vi "Selectively clear model queue.vi"(7 "Queue clearing option":T2, 8 "error in (no error)":errorcluster, 11 "State(s) to look for [One per line]":string) -> (0 "error out":errorcluster, 3 "Cleared states":T1[](array[typedef]))   [LabVIEW 2018]
doc: "Get the queue reference and acts upon what is stored in it according to the \"Queue clearing option\" input.\n\nThe \"State(s) to look for\" input is the same format as the input for the \"Enqueue many states to controller\" VI. Meaning that it should be case-insensitive strings that name case(s), one per line, that pertain to the selected clearing option.\n\n\"Clear entire queue\" removes all pending states.\n\"Clear all that match\" removes all states, then re-queues states that don't match any of the ones in the input list.\n\"Clear all that don't match\" removes all states, then re-queues states that match one of the ones in the input list.\n\"Clear one of each match\" removes all states, then re-queues states that don't match the input list, but the input list only removes exactly one state per matching entry. This can be used to remove the first state that matches but leave the rest."
uses:
  Selective queue clearing methods.ctl
  Model queue data.ctl
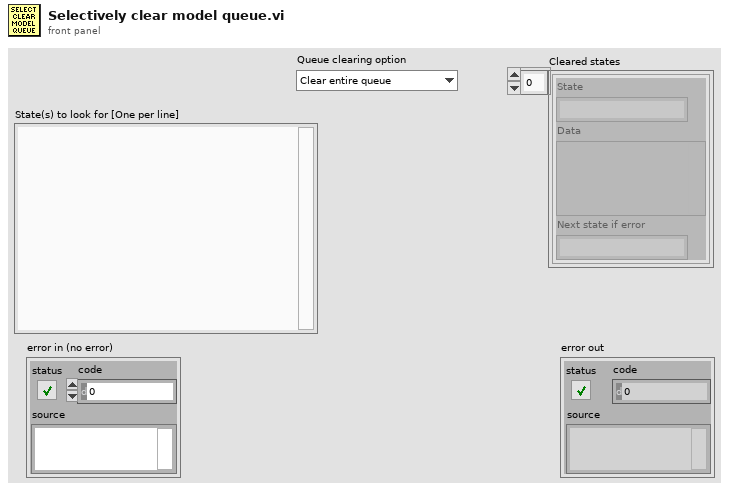
[diagram p1: front panel]
types:
  T1 = typedef "Model queue data.ctl" = cluster{"State":string, "Data":variant, "Next state if error":string}
  T2 = typedef "Selective queue clearing methods.ctl" = enum16{"Clear entire queue", "Clear all that match", "Clear all that don't match", "Clear one of each match"}
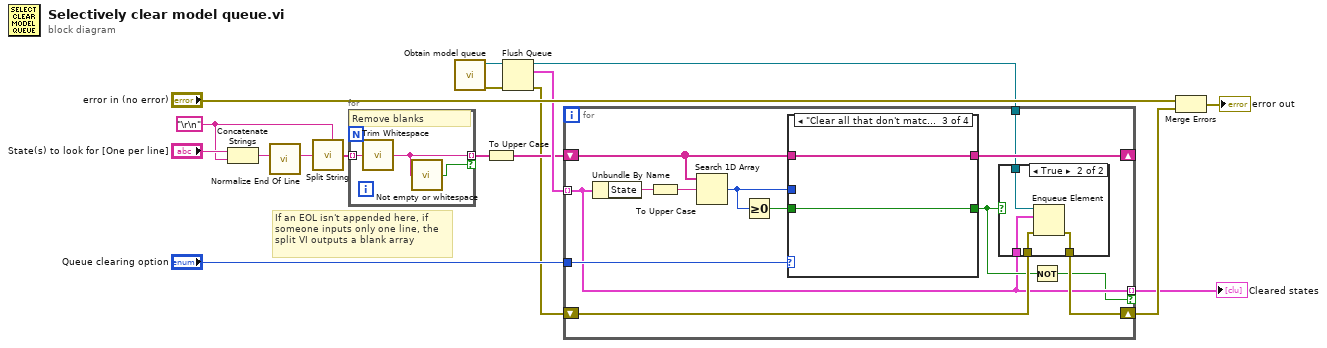
[diagram p0: block diagram]
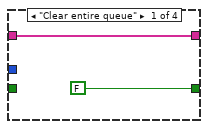
[diagram p3: hidden frame]
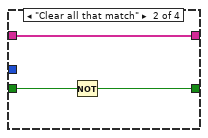
[diagram p4: hidden frame]
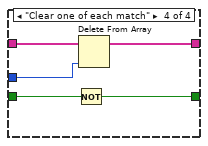
[diagram p5: hidden frame]
diagram:
  w9 = "\r\n"
  # "If an EOL isn't appended here, if someone inputs only one line, the split VI outputs a blank array"
  n1 = Concatenate Strings("State(s) to look for [One per line]", w9) -> (w10:string)
  n2 = call <vilib>:"Normalize End Of Line.vi"("string in"=w10) -> ("string out"=w8:string)  [unwired: 7 in]
  n3 = call <vilib>:"Split String.vi"("Split Pattern"=w9, "Input String"=w8) -> ("Split String"=w12:string[])  [unwired: 5 in]
  n4 = for {
    tunnel: w12 -> [w20] mode=indexing
    tunnel: [w19] -> w7 mode=indexing if=w18
    # "Remove blanks"
    n5 = call <vilib>:"Trim Whitespace.vi"("string"=w20) -> ("trimmed string"=w19:string)  [unwired: 1 in]
    n6 = call <userlib>:"Not empty or whitespace.vi"("String"=w19) -> ("Not empty or all whitespace"=w18:bool)  [unwired: 4 in]
  }
  n7 = call "Obtain model queue.vi"() -> ("error out"=w15:errorcluster, "Model loop queue"=w14:refnum<queue>)  [unwired: 10 in]
  n8 = To Upper Case(1:w7) -> (0:w6:string[])
  n9 = Flush Queue(queue=w14, error in (no error)=w15) -> (queue out=w4:refnum<queue>, remaining elements=w13:T1[], error out=w3:errorcluster)
  n10 = for {
    tunnel: w13 -> [w22] mode=indexing
    shift-right: [w29] -> _
    shift-left: w6 -> [w31]
    tunnel: "Queue clearing option" -> [w30]
    tunnel: w4 -> [w26]
    shift-right: [w24] -> w2
    shift-left: w3 -> [w25]
    tunnel: [w22] -> w1 mode=indexing if=w21
    n11 = Unbundle By Name(w22) -> ("State"=w33:string)
    n12 = To Upper Case(1:w33) -> (0:w32:string)
    n13 = Search 1D Array(1D array=w31, element=w32) -> (index of element=w27:i32)  [unwired: 1 in]
    n14 = Greater Or Equal To 0?(x=w27) -> (x >= 0?=w28:bool)
    n15 = case shown="\"Clear all that don't match\"" w30 {
      tunnel: w31 -> [w40 w41 w44 w50]
      tunnel: [w40 w41 w44 w48] -> w29
      tunnel: [FALSE w42 w45 w46] -> w23
      tunnel: w28 -> [_ w43 w45 w47]
      tunnel: w27 -> [_ _ _ w49]
      frame "Clear entire queue" {
      }
      frame "Clear all that match" {
        n16 = Not(x=w43) -> (.not. x?=w42:bool)
      }
      frame "Clear all that don't match" {
      }
      frame "Clear one of each match" {
        n17 = Not(x=w47) -> (.not. x?=w46:bool)
        n18 = Delete From Array(array=w50, index=w49) -> (array with subset deleted=w48:string[])  [unwired: 1 in, 1 out]
      }
    }
    n19 = case shown="True" w23 {
      tunnel: w26 -> [_ w38]
      tunnel: w22 -> [_ w37]
      tunnel: w25 -> [w34 w36]
      tunnel: [w34 w35] -> w24
      frame False {
      }
      frame True {
        n20 = Enqueue Element(queue=w38, element=w37, error in (no error)=w36) -> (error out=w35:errorcluster)  [unwired: 1 in, 2 out]
      }
    }
    n21 = Not(x=w23) -> (.not. x?=w21:bool)
  }
  "Cleared states" <- w1
  n22 = Merge Errors("error in (no error)", w2) -> (→"error out":errorcluster)
